vi "Get LowLimit.vi"(8 "error in":errorcluster, 11 "DOMAIN in":refnum<class "DOMAIN.lvclass">) -> (0 "error out":errorcluster, 1 "Set?":bool, 2 "LowLimit":string, 3 "DOMAIN out":refnum<class "DOMAIN.lvclass">)   [LabVIEW 2024, in "Electronic Datasheet.lvlib" / "DOMAIN.lvclass"]
uses:
  DOMAIN.lvclass
  Electronic Datasheet.lvlib
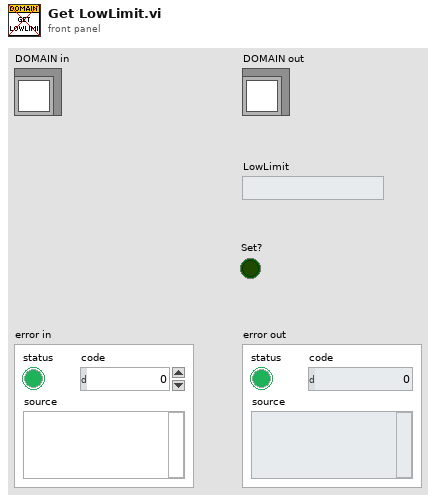
[diagram p1: front panel]
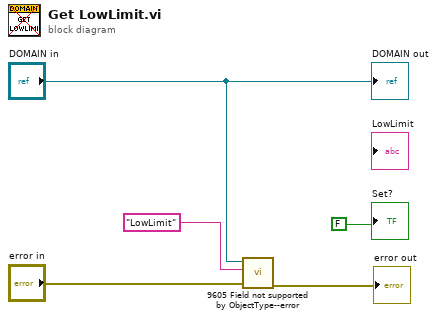
[diagram p0: block diagram]
diagram:
  n1 = call "9605 Field not supported by ObjectType--error.vi"("error in"="error in", "Field Name"="LowLimit" ("Field name"), "Object Type Base"="DOMAIN in") -> ("error out"=→"error out":errorcluster)  [unwired: 8 in]
  "DOMAIN out" <- "DOMAIN in"
  "Set?" <- FALSE ("Set?")
